vi "XIPIN_AXI_MMU_2_1.vi"   [LabVIEW 2017]
doc: "The AXI MMU IP provides addres range decoding and remapping services for AXI Interconnect.\n------------------------------------\n<b>Need License</b> : No\n<b>Interface</b> : AXI4"
uses:
  <vilib>/rvi/XilinxIP/XIPIN_XNode/niFpgaXIPIN.xnode
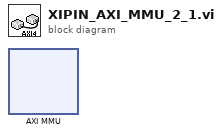
[diagram p0: block diagram]
diagram:
  n1 = xnode ("AXI MMU")() -> ()
